vi "Read Artifact Days.vi"(8 "error in (no error)":errorcluster, 11 "CI Project in":refnum<class "CI Project.lvclass">) -> (0 "error out":errorcluster, 2 "Artifact Days":i32=1 min=1, 3 "CI Project out":refnum<class "CI Project.lvclass">)   [LabVIEW 2014, in "CI Project.lvclass"]
uses:
  CI Project.lvclass
  CI Project.lvclass/CI Project.ctl
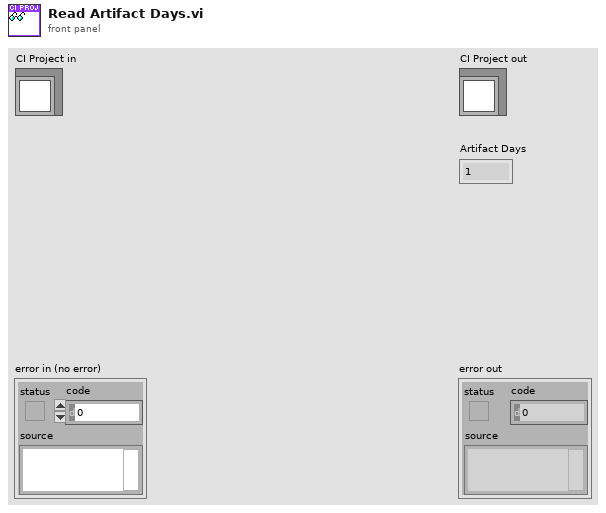
[diagram p1: front panel]
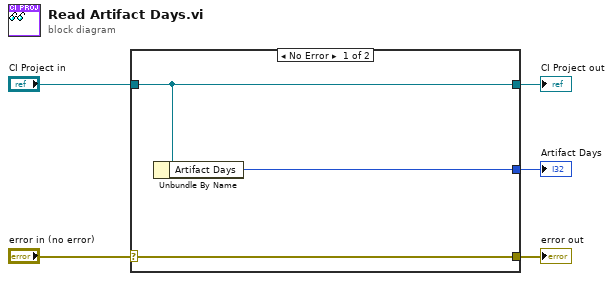
[diagram p0: block diagram]
diagram:
  n1 = case shown="No Error" "error in (no error)" {
    selector: "error in (no error)" -> [w8 w9]
    tunnel: [w8 w9] -> w4
    tunnel: [w7 w10] -> w2
    tunnel: "CI Project in" -> [w7 w10]
    tunnel: [w6 _] -> w1
    frame No Error {
      n2 = Unbundle By Name(w7) -> ("Artifact Days"=w6:i32)
    }
    frame Error {
    }
  }
  "error out" <- w4
  "CI Project out" <- w2
  "Artifact Days" <- w1
